vi "Predict Cuboid GB Dimensions.vi"(9 "Mutual Viewing Angle":dbl[](array[numeric])=[1.0, 0.0, 0.0], 10 "Tolerance":dbl=0.001, 11 "Grain Boundary Macro Definition":T3={"Grain 1 Orientation"=[1.0, 0.6019417241891012, 0.029651947654046266], "Grain 2 Orientation"=[1.0, 0.730727623275494, 0.2205637301176], "Twist Angle (Deg)"=0.0}) -> (1 "Height Error":dbl, 2 "Width Error":dbl, 3 "Suggested Cuboid Dimensions (proportional)":T1)   [LabVIEW 2010]
uses:
  <vilib>/Analysis/Matrix/Datatypes/RealMatrix.ctl
  <vilib>/Analysis/baseanly.llb/Real A x B.vi
  <vilib>/Analysis/baseanly.llb/A x Vector.vi
  <vilib>/Analysis/NI_AALPro.lvlib
  <vilib>/Analysis/NI_AALBase.lvlib
  <vilib>/Analysis/Matrix/NI_Matrix.lvlib
panel:
  out "System Numeric Array":dbl[][](array[numeric])
  out "Grain 2 Height":dbl
  out "Grain 1 Height":dbl
  out "Grain 2 Width":dbl
  out "Grain 1 Width":dbl
  in  "Lattice Parameter":dbl=6.615785553057252
  out "Try this height":dbl
  out "Try this width":dbl
  out "Suggested X 2":dbl
  out "Suggested Y 2":dbl
  out "Suggested Grain 2 Length":dbl
  out "Suggested Grain 1 Length":dbl
  out "Suggested Y":dbl
  out "Suggested X":dbl
  out "Grain A":T2
  out "Grain B":T2
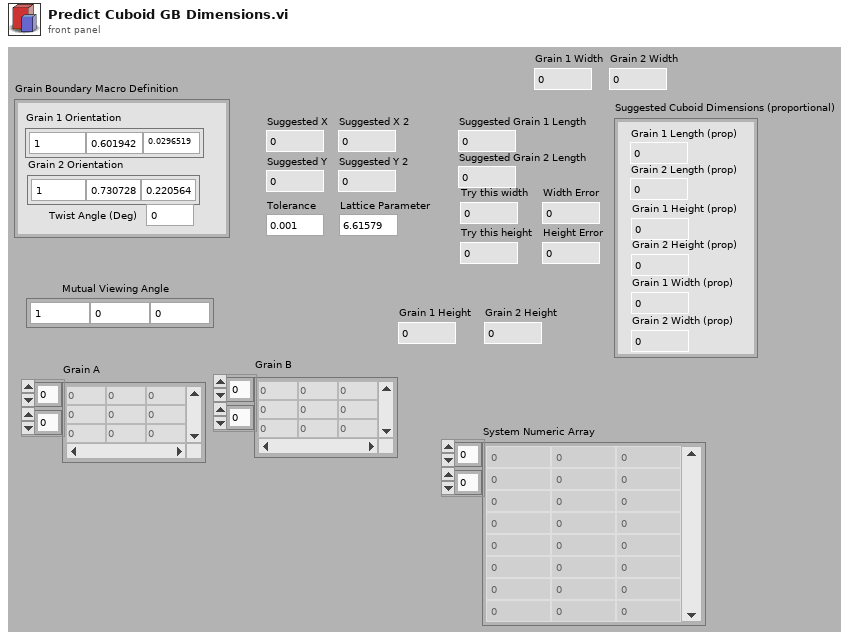
[diagram p1: front panel]
types:
  T1 = cluster{"Grain 1 Length (prop)":dbl, "Grain 2 Length (prop)":dbl, "Grain 1 Height (prop)":dbl, "Grain 2 Height (prop)":dbl, "Grain 1 Width (prop)":dbl, "Grain 2 Width (prop)":dbl}
  T2 = typedef "NI_Matrix.lvlib/RealMatrix.ctl" = dbl[][]
  T3 = cluster{"Grain 1 Orientation":dbl[], "Grain 2 Orientation":dbl[], "Twist Angle (Deg)":dbl}
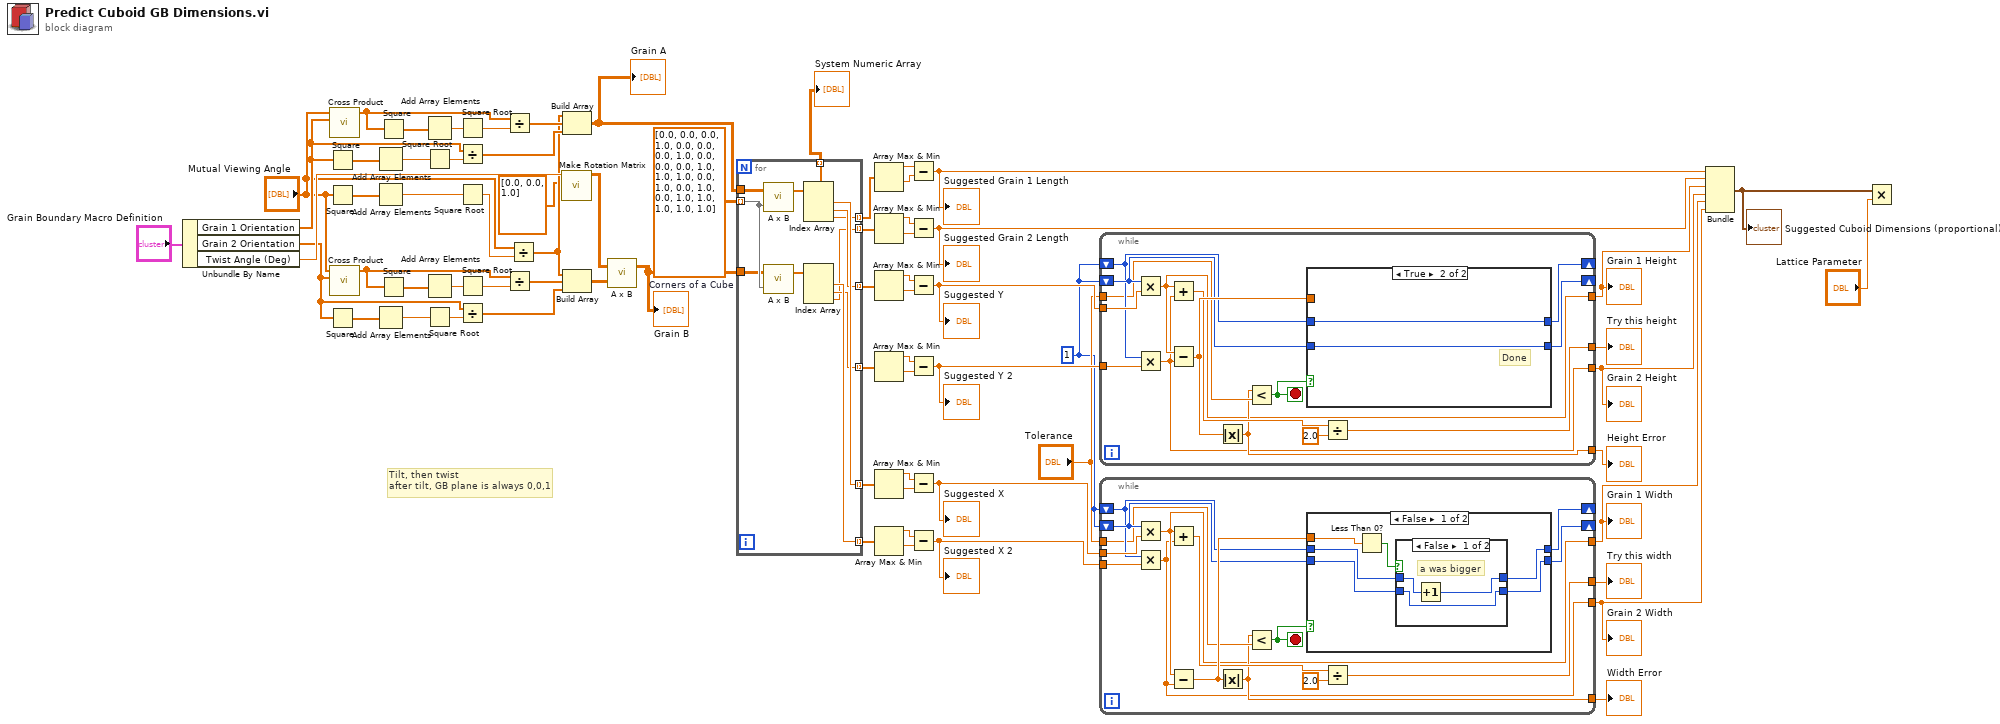
[diagram p0: block diagram]
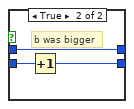
[diagram p2: hidden frame]
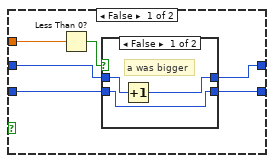
[diagram p4: hidden frame]
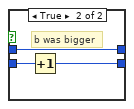
[diagram p5: hidden frame]
diagram:
  w62 = dbl[][] [[0.0, 0.0, 0.0], [1.0, 0.0, 0.0], [0.0, 1.0, 0.0], [0.0, 0.0, 1.0], [1.0, 1.0, 0.0], [1.0, 0.0, 1.0], [0.0, 1.0, 1.0], [1.0, 1.0, 1.0]]  # Corners of a Cube
  w36 = 1
  # "Tilt, then twist\nafter tilt, GB plane is always 0,0,1"
  n1 = Unbundle By Name("Grain Boundary Macro Definition") -> ("Grain 1 Orientation"=w23:dbl[], "Grain 2 Orientation"=w3:dbl[], "Twist Angle (Deg)"=w64:dbl)
  n2 = Square(x=w23) -> (x^2=w22:dbl[])
  n3 = Square(x="Mutual Viewing Angle") -> (x^2=w18:dbl[])
  n4 = Square(x=w3) -> (x^2=w4:dbl[])
  n5 = call <vilib>:"Cross Product.vi"("B Vector"=w23, "A Vector"="Mutual Viewing Angle") -> ("Cross Product"=w12:dbl[])  [unwired: 8 in, 1 out]
  n6 = call <vilib>:"Cross Product.vi"("B Vector"=w3, "A Vector"="Mutual Viewing Angle") -> ("Cross Product"=w8:dbl[])  [unwired: 8 in, 1 out]
  n7 = Add Array Elements(numeric array=w22) -> (sum=w21:dbl)
  n8 = Add Array Elements(numeric array=w18) -> (sum=w19:dbl)
  n9 = Add Array Elements(numeric array=w4) -> (sum=w5:dbl)
  n10 = Square(x=w12) -> (x^2=w14:dbl[])
  n11 = Square(x=w8) -> (x^2=w10:dbl[])
  n12 = Add Array Elements(numeric array=w14) -> (sum=w13:dbl)
  n13 = Square Root(x=w21) -> (sqrt(x)=w20:dbl)
  n14 = Add Array Elements(numeric array=w10) -> (sum=w9:dbl)
  n15 = Square Root(x=w5) -> (sqrt(x)=w2:dbl)
  n16 = Square Root(x=w13) -> (sqrt(x)=w11:dbl)
  n17 = Divide(x=w23, y=w20) -> (x/y=w70:dbl[])
  n18 = Square Root(x=w19) -> (sqrt(x)=w15:dbl)
  n19 = Square Root(x=w9) -> (sqrt(x)=w7:dbl)
  n20 = Divide(x=w3, y=w2) -> (x/y=w66:dbl[])
  n21 = Divide(x=w12, y=w11) -> (x/y=w69:dbl[])
  n22 = Divide(x=w8, y=w7) -> (x/y=w68:dbl[])
  n23 = Divide(x="Mutual Viewing Angle", y=w15) -> (x/y=w17:dbl[])
  n24 = call "Make Rotation Matrix.vi"("Rotation Axis"=dbl[] [0.0, 0.0, 1.0], "Rotation Angle (Degree)"=w64) -> ("Rotation Matrix"=w67:T2)  [unwired: 9 in]
  n25 = Build Array(w17, w69, w70) -> (w61:T2)
  "Grain A" <- w61
  n26 = Build Array(w17, w68, w66) -> (w65:T2)
  n27 = call-poly <vilib>:"A x B.vi"("B"=w65, "A"=w67) -> ("A x B"=w60:T2)  [unwired: 1 out]
  "Grain B" <- w60
  n28 = for {
    tunnel: w62 -> [w80] mode=indexing
    tunnel: w61 -> [w81]
    tunnel: w60 -> [w79]
    tunnel: [w77] -> w53 mode=indexing
    tunnel: [w76] -> w52 mode=indexing
    tunnel: [w75] -> w51 mode=indexing
    tunnel: [w74] -> w44 mode=indexing
    tunnel: [w73] -> w43 mode=indexing
    tunnel: [w72] -> w42 mode=indexing
    tunnel: [w71] -> w1 mode=indexing
    n29 = call-poly <vilib>:"A x B.vi"("Vector"=w80, "A"=w81) -> ("A x Vector"=w71:dbl[])  [unwired: 1 out]
    n30 = call-poly <vilib>:"A x B.vi"("Vector"=w80, "A"=w79) -> ("A x Vector"=w78:dbl[])  [unwired: 1 out]
    n31 = Index Array(array=w71) -> (element #1=w77:dbl, element #2=w76:dbl, element #3=w75:dbl)  [unwired: 3 in]
    n32 = Index Array(array=w78) -> (element #1=w74:dbl, element #2=w73:dbl, element #3=w72:dbl)  [unwired: 3 in]
  }
  "System Numeric Array" <- w1
  n33 = Array Max & Min(array=w51) -> (max value=w55:dbl, min value=w54:dbl)  [unwired: 2 out]
  n34 = Array Max & Min(array=w42) -> (max value=w49:dbl, min value=w50:dbl)  [unwired: 2 out]
  n35 = Array Max & Min(array=w52) -> (max value=w56:dbl, min value=w57:dbl)  [unwired: 2 out]
  n36 = Array Max & Min(array=w43) -> (max value=w48:dbl, min value=w47:dbl)  [unwired: 2 out]
  n37 = Array Max & Min(array=w53) -> (max value=w59:dbl, min value=w58:dbl)  [unwired: 2 out]
  n38 = Array Max & Min(array=w44) -> (max value=w45:dbl, min value=w46:dbl)  [unwired: 2 out]
  n39 = Subtract(x=w55, y=w54) -> (x-y=w34:dbl)
  "Suggested Grain 1 Length" <- w34
  n40 = Subtract(x=w49, y=w50) -> (x-y=w33:dbl)
  "Suggested Grain 2 Length" <- w33
  n41 = Subtract(x=w56, y=w57) -> (x-y=w41:dbl)
  "Suggested Y" <- w41
  n42 = Subtract(x=w48, y=w47) -> (x-y=w40:dbl)
  "Suggested Y 2" <- w40
  n43 = Subtract(x=w59, y=w58) -> (x-y=w38:dbl)
  "Suggested X" <- w38
  n44 = Subtract(x=w45, y=w46) -> (x-y=w37:dbl)
  "Suggested X 2" <- w37
  n45 = while {
    shift-right: [w91] -> _
    shift-left: w36 -> [w92]
    shift-right: [w89] -> _
    shift-left: w36 -> [w90]
    tunnel: w41 -> [w96]
    tunnel: w40 -> [w95]
    tunnel: [w85] -> w32
    tunnel: "Tolerance" -> [w88]
    tunnel: [w84] -> w35
    tunnel: [w83] -> w28
    tunnel: [w82] -> w27
    stop <- w94 stop-if-true
    n46 = Multiply(x=w92, y=w96) -> (x*y=w83:dbl)
    n47 = Multiply(x=w90, y=w95) -> (x*y=w82:dbl)
    n48 = Add(x=w83, y=w82) -> (x+y=w86:dbl)
    n49 = Subtract(x=w83, y=w82) -> (x-y=w93:dbl)
    n50 = Absolute Value(x=w93) -> (abs(x)=w84:dbl)
    n51 = Less?(x=w84, y=w88) -> (x < y?=w94:bool)
    n52 = case shown="True" w94 {
      tunnel: w93 -> [w102 _]
      tunnel: w92 -> [w101 w110]
      tunnel: [w100 w110] -> w91
      tunnel: w90 -> [w99 w109]
      tunnel: [w98 w109] -> w89
      frame False {
        n53 = Less Than 0?(x=w102) -> (x < 0?=w97:bool)
        n54 = case shown="False" w97 {
          tunnel: w101 -> [w103 w108]
          tunnel: [w103 w107] -> w100
          tunnel: w99 -> [w105 w106]
          tunnel: [w104 w106] -> w98
          frame False {
            # "a was bigger"
            n55 = Increment(x=w105) -> (x+1=w104:i32)
          }
          frame True {
            # "b was bigger"
            n56 = Increment(x=w108) -> (x+1=w107:i32)
          }
        }
      }
      frame True {
        # "Done"
      }
    }
    n57 = Divide(x=w86, y=2.0) -> (x/y=w85:dbl)
  }
  "Try this height" <- w32
  "Height Error" <- w35
  "Grain 1 Height" <- w28
  "Grain 2 Height" <- w27
  n58 = while {
    shift-right: [w120] -> _
    shift-left: w36 -> [w121]
    shift-right: [w118] -> _
    shift-left: w36 -> [w119]
    tunnel: w38 -> [w125]
    tunnel: w37 -> [w124]
    tunnel: [w114] -> w30
    tunnel: "Tolerance" -> [w117]
    tunnel: [w113] -> w31
    tunnel: [w112] -> w26
    tunnel: [w111] -> w25
    stop <- w123 stop-if-true
    n59 = Multiply(x=w121, y=w125) -> (x*y=w112:dbl)
    n60 = Multiply(x=w119, y=w124) -> (x*y=w111:dbl)
    n61 = Add(x=w112, y=w111) -> (x+y=w115:dbl)
    n62 = Subtract(x=w112, y=w111) -> (x-y=w122:dbl)
    n63 = Absolute Value(x=w122) -> (abs(x)=w113:dbl)
    n64 = Less?(x=w113, y=w117) -> (x < y?=w123:bool)
    n65 = case shown="False" w123 {
      tunnel: w122 -> [w131 _]
      tunnel: w121 -> [w130 w139]
      tunnel: [w129 w139] -> w120
      tunnel: w119 -> [w128 w138]
      tunnel: [w127 w138] -> w118
      frame False {
        n66 = Less Than 0?(x=w131) -> (x < 0?=w126:bool)
        n67 = case shown="False" w126 {
          tunnel: w130 -> [w132 w137]
          tunnel: [w132 w136] -> w129
          tunnel: w128 -> [w134 w135]
          tunnel: [w133 w135] -> w127
          frame False {
            # "a was bigger"
            n68 = Increment(x=w134) -> (x+1=w133:i32)
          }
          frame True {
            # "b was bigger"
            n69 = Increment(x=w137) -> (x+1=w136:i32)
          }
        }
      }
      frame True {
        # "Done"
      }
    }
    n70 = Divide(x=w115, y=2.0) -> (x/y=w114:dbl)
  }
  "Try this width" <- w30
  "Width Error" <- w31
  "Grain 1 Width" <- w26
  "Grain 2 Width" <- w25
  n71 = Bundle(w34, w33, w28, w27, w26, w25) -> (w24:cluster{dbl, dbl, dbl, dbl, dbl, dbl})  [unwired: 1 in]
  "Suggested Cuboid Dimensions (proportional)" <- w24
  n72 = Multiply(x=w24, y="Lattice Parameter") -> ()  [unwired: 1 out]
